vi "Write Read Example.vi"() -> ()   [LabVIEW 2014]
panel:
  out "error out":errorcluster
  out "String read":string
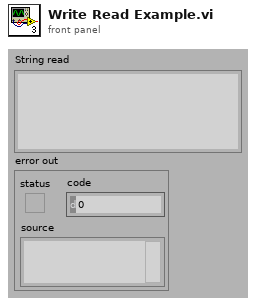
[diagram p1: front panel]
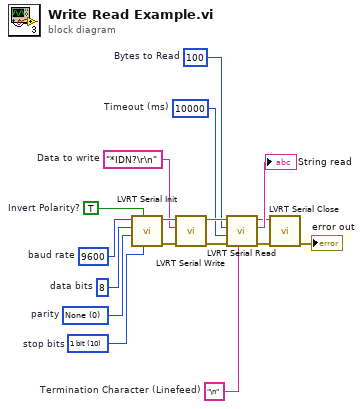
[diagram p0: block diagram]
diagram:
  w1 = u16 10 items=["1 bit"=10, "1.5 bits"=15, "2 bits"=20]  # stop bits
  w2 = u16 0 items=["None", "Odd", "Even", "Mark", "Space"]  # parity
  w3 = u16 8  # data bits
  w4 = TRUE  # Invert Polarity?
  w5 = "\n"  # Termination Character (Linefeed)
  w6 = 10000  # Timeout (ms)
  w11 = u32 100  # Bytes to Read
  w15 = "*IDN?\r\n"  # Data to write
  w17 = u32 9600  # baud rate
  n1 = call "LVRT Serial Init.vi"("stop bits (10: 1 bit)"=w1, "Invert Polarity?"=w4, "parity (0:none)"=w2, "data bits (8)"=w3, "baud rate (9600)"=w17) -> ("error out"=w14:errorcluster, "FPGA Main Reference Out"=w16:refnum<k20>)  [unwired: 1 in, 4 out]
  n2 = call "LVRT Serial Write.vi"("error in (no error)"=w14, "String"=w15, "FPGA Main Ref"=w16) -> ("error out"=w13:errorcluster, "FPGA Main Ref Out"=w12:refnum<k20>)  [unwired: 7 out]
  n3 = call "LVRT Serial Read.vi"("Termination Character (Linefeed)"=w5, "error in (no error)"=w13, "Timeout (ms) (-1: no timeout)"=w6, "Bytes to Read"=w11, "FPGA Main Ref"=w12) -> ("error out"=w8:errorcluster, "String"=→"String read":string, "FPGA Main Ref Out"=w9:refnum<k20>)  [unwired: 4 out]
  n4 = call "LVRT Serial Close.vi"("error out"=w8, "FPGA Main Ref"=w9) -> ("error out"=→"error out":errorcluster)  [unwired: 9 out]
